vi "KE487_Test.vi"(8 "error in (no error)":errorcluster, 11 "KE487 in":refnum<class "KE487.lvclass">) -> (0 "error out":errorcluster, 3 "KE487 out":refnum<class "KE487.lvclass">)   [LabVIEW 2013, in "KE487.lvclass"]
uses:
  KE487.lvclass
  <vilib>/Platform/TimedLoop/XDataNode/timing_clust.ctl
  <vilib>/Platform/TimedLoop/XDataNode/nitl_modes.ctl
  <vilib>/Platform/TimedLoop/XDataNode/wakeup.ctl
  <vilib>/platform/TimedLoop/XDataNode/XDataNode.xnode
  <vilib>/Platform/TimedLoop/XDataNode/XDNodeRunTimeDep.lvlib
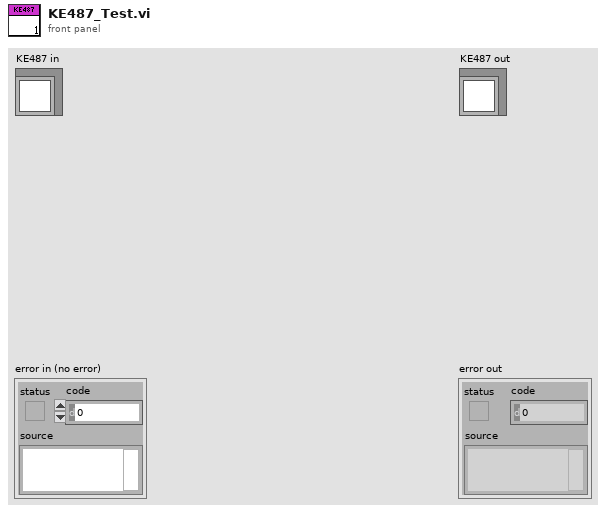
[diagram p1: front panel]
types:
  T1 = typedef "XDNodeRunTimeDep.lvlib/timing_clust.ctl" = cluster{"Expected End [f-1]":u64, "Actual End [f-1]":u64, "Finished Late? [f-1]":bool, "Expected End [i-1]":u64, "Actual End [i-1]":u64, "Finished Late? [i-1]":bool, "Expected Start [i]":u64, "Actual Start [i]":u64, "Expected Start [f]":u64, "Actual Start [f]":u64, "Source Name":string, "Structure Name":string, "Period":i64, "Deadline":i64, "Offset":i64, "Start":i64, "Priority":i32, "Timeout":i32, "Mode":T2, "Wakeup Reason":T3, "Error":errorcluster, "Source Type":string, "Secondary Source Type":string, "Global End Time":u64, "Global Start Time":u64, "Frame Duration":u64, "Iteration Duration":u64, "Assigned CPU":i32, "I/O Scan Engine Mode":u32}
  T2 = typedef "XDNodeRunTimeDep.lvlib/nitl_modes.ctl" = enum32{"No Change", "Process missed periods, maintain original phase", "Discard missed periods, maintain original phase", "Process missed periods, ignore original phase", "Discard missed periods, ignore original phase"}
  T3 = typedef "XDNodeRunTimeDep.lvlib/wakeup.ctl" = enum32{"Normal", "Aborted", "Asynchronous wakeup", "Timing source error", "Timed loop error", "Timeout"}
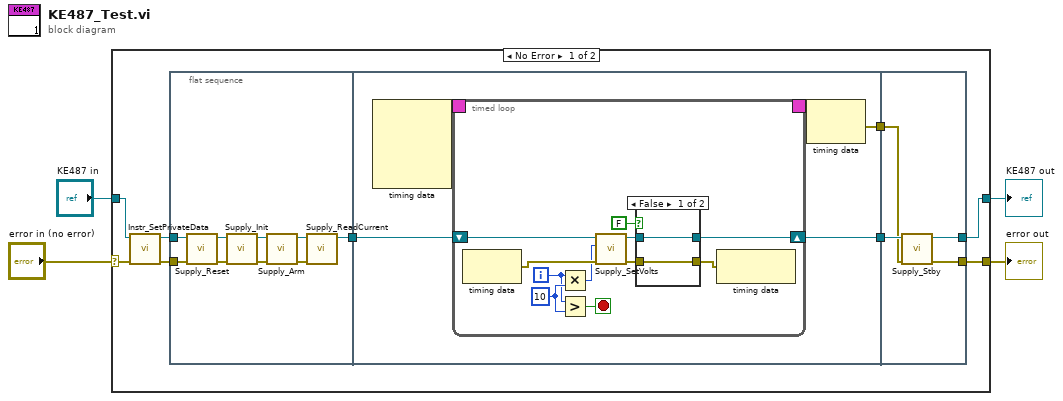
[diagram p0: block diagram]
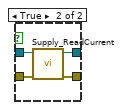
[diagram p2: hidden frame]
diagram:
  n1 = case shown="No Error" "error in (no error)" {
    selector: "error in (no error)" -> [w7 w58]
    tunnel: [w6 w58] -> w3
    tunnel: [w5 w57] -> w1
    tunnel: "KE487 in" -> [w8 w57]
    frame No Error {
      n2 = call-dynamic "Instr_SetPrivateData.vi"("error in (no error)"=w7, "KE487 in"=w8) -> ("error out"=w10:errorcluster, "KE487 out"=w9:refnum<class "KE487.lvclass">)  [unwired: 8 in]
      n3 = flat-sequence {
        tunnel: w10 -> [w17]
        tunnel: w9 -> [w16]
        tunnel: [w14] -> w13
        tunnel: w13 -> [w27]
        tunnel: [w26] -> w12
        tunnel: [w23] -> w11
        tunnel: [w54] -> w6
        tunnel: w12 -> [w55]
        tunnel: w11 -> [w56]
        tunnel: [w53] -> w5
        frame #0 {
          n4 = call-dynamic "Supply_Reset.vi"("error in (no error)"=w17, "SupplyControl in"=w16) -> ("error out"=w21:errorcluster, "SupplyControl out"=w15:refnum<class "KE487.lvclass">)  [unwired: 8 in]
          n5 = call-dynamic "Supply_Init.vi"("error in (no error)"=w21, "SupplyControl in"=w15) -> ("error out"=w20:errorcluster, "SupplyControl out"=w22:refnum<class "KE487.lvclass">)  [unwired: 8 in]
          n6 = call-dynamic "Supply_Arm.vi"("error in (no error)"=w20, "SupplyControl in"=w22) -> ("error out"=w18:errorcluster, "SupplyControl out"=w19:refnum<class "KE487.lvclass">)  [unwired: 8 in]
          n7 = call-dynamic "Supply_ReadCurrent.vi"("error in (no error)"=w18, "SupplyControl in"=w19) -> ("SupplyControl out"=w14:refnum<class "KE487.lvclass">)  [unwired: 7 in, 2 out]
        }
        frame #1 {
          n8 = node-c288() -> (w25:T1)  [unwired: 4 in]
          n9 = timed-loop {
            timing: w25 -> [_]
            timing-out: [_] -> w24
            shift-right: [w30] -> w23
            shift-left: w27 -> [w36]
            i -> [w34]
            stop <- w33 stop-if-true
            w35 = 10
            n10 = node-c288() -> (w38:errorcluster)  [unwired: 1 in]
            n11 = Multiply(x=w34, y=w35) -> (x*y=w37:i32)
            n12 = Greater?(x=w34, y=w35) -> (0:w33:bool)
            n13 = call-dynamic "Supply_SetVolts.vi"("error in (no error)"=w38, "Volts IN [V]"=w37, "KE487 in"=w36) -> ("error out"=w32:errorcluster, "KE487 out"=w31:refnum<class "KE487.lvclass">)  [unwired: 6 in, 1 out]
            n14 = case shown="False" FALSE {
              tunnel: w32 -> [w40 w44]
              tunnel: w31 -> [w39 w43]
              tunnel: [w39 w42] -> w30
              tunnel: [w40 w41] -> w29
              frame False {
              }
              frame True {
                n15 = call-dynamic "Supply_ReadCurrent.vi"("error in (no error)"=w44, "SupplyControl in"=w43) -> ("error out"=w41:errorcluster, "SupplyControl out"=w42:refnum<class "KE487.lvclass">)  [unwired: 7 in, 1 out]
              }
            }
            n16 = node-c288(w29) -> ()  [unwired: 1 out]
          }
          n17 = node-c288(w24) -> (w26:errorcluster)
        }
        frame #2 {
          n18 = call-dynamic "Supply_Stby.vi"("error in (no error)"=w55, "SupplyControl in"=w56) -> ("error out"=w54:errorcluster, "SupplyControl out"=w53:refnum<class "KE487.lvclass">)  [unwired: 8 in]
        }
      }
    }
    frame Error {
    }
  }
  "error out" <- w3
  "KE487 out" <- w1
